vi "Counter - Read Pulse Duty Cycle and Frequency (Continuous).vi"() -> ()   [LabVIEW 2017]
doc: "该范例演示了如何基于外部时钟进行脉冲测量，以获得频率和占空比。\n\nNI的X系列和第二代NI CompactDAQ设备中增加了脉冲测量功能。\n\n关于将信号连接至DAQ设备的方法，可参考设备文档。"
uses:
  <vilib>/Utility/error.llb/DialogType.ctl
  <vilib>/DAQmx/read.llb/DAQmx Read (Counter 1D Pulse Freq 1 Chan NSamp).vi
  <vilib>/DAQmx/create/channels.llb/DAQmx Create Channel (CI-Pulse Freq).vi
  <vilib>/DAQmx/configure/timing.llb/DAQmx Timing (Sample Clock).vi
  <vilib>/DAQmx/miscellaneous.llb/DAQmx Fill In Error Info.vi
  <resource>/objmgr/daqmx.rc
panel:
  out "数据数组":cluster{"占空比":dbl, "频率":dbl}[](array[cluster])
  in  "采样率":dbl=1000.0
  in  "外部时钟源":tag="PFI0"
  in  "最小频率":dbl=2.0 format="%0.6f"
  in  "最大频率":dbl=100.0 format="%0.6f"
  in  "脉冲频率接线端":tag="PFI9"
  in  "停止":bool
  in  "每次循环采样数":i32=1000
  in  "计数器":tag="Dev1/ctr0"
  # "通道设置"
  # "采集数据"
  # "定时设置"
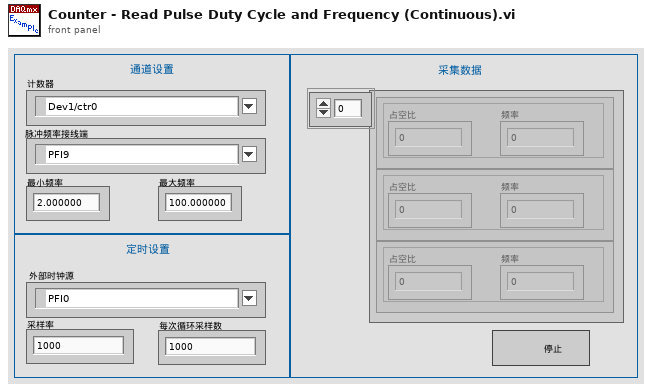
[diagram p1: front panel]
types:
  T1 = typedef "DialogType.ctl" = u16
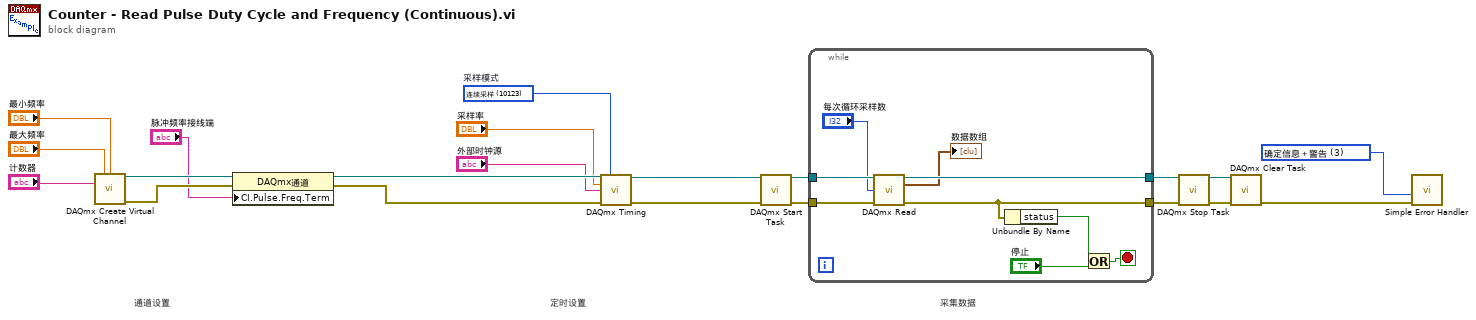
[diagram p0: block diagram]
diagram:
  w1 = T1 3 items=["无对话框", "确定信息", "继续或停止信息", "确定信息＋警告", "继续/停止＋警告"] ("对话框类型（确定信息：1）")
  w21 = 10123 items=["有限采样"=10178, "连续采样"=10123, "硬件定时单点"=12522]  # 采样模式
  # "采集数据"
  # "定时设置"
  # "通道设置"
  n1 = call-poly <vilib>:"DAQmx Create Virtual Channel.vi"("maximum value"="最大频率", "minimum value"="最小频率", "counter"="计数器") -> ("task out"=w12:refnum<k21>, "error out"=w11:errorcluster)  [unwired: 11 in]
  n2 = property class="DAQmx通道"(reference=w12, error in=w11, "CI.Pulse.Freq.Term"="脉冲频率接线端") -> (reference out=w19:refnum<k21>, error out=w20:errorcluster)
  n3 = call-poly <vilib>:"DAQmx Timing.vi"("task/channels in"=w19, "sample mode"=w21, "rate"="采样率", "source"="外部时钟源", "error in"=w20) -> ("task out"=w14:refnum<k21>, "error out"=w13:errorcluster)  [unwired: 9 in]
  n4 = call <vilib>:"DAQmx Start Task.vi"("task/channels in"=w14, "error in"=w13) -> ("task out"=w18:refnum<k21>, "error out"=w17:errorcluster)  [unwired: 12 in]
  n5 = while {
    tunnel: w18 -> [w30]
    tunnel: w17 -> [w29]
    tunnel: [w26] -> w2
    tunnel: [w27] -> w3
    stop <- w28 stop-if-true
    n6 = call-poly <vilib>:"DAQmx Read.vi"("task/channels in"=w30, "number of samples per channel"="每次循环采样数", "error in"=w29) -> ("task out"=w27:refnum<k21>, "data"=→"数据数组":cluster{"duty cycle":dbl, "frequency":dbl}[], "error out"=w26:errorcluster)  [unwired: 10 in]
    n7 = Unbundle By Name(w26) -> ("status"=w25:bool)
    n8 = Or(x=w25, y="停止") -> (x .or. y?=w28:bool)
  }
  n9 = call <vilib>:"DAQmx Stop Task.vi"("task/channels in"=w3, "error in"=w2) -> ("task out"=w5:refnum<k21>, "error out"=w4:errorcluster)  [unwired: 12 in]
  n10 = call <vilib>:"DAQmx Clear Task.vi"("task in"=w5, "error in"=w4) -> ("error out"=w16:errorcluster)  [unwired: 13 in]
  n11 = call <vilib>:"Simple Error Handler.vi"("type of dialog (OK msg:1)"=w1, "error in (no error)"=w16) -> ()  [unwired: 3 in, 5 out]
